vi "Append Strings to Log Control.vi"(8 "エラー入力 (エラーなし)":errorcluster, 10 "Appending Strings":string, 11 "Result Log Reference":refnum<vi>) -> (0 "エラー出力":errorcluster, 3 "Result Log Reference Out":refnum<vi>)   [LabVIEW 2020]
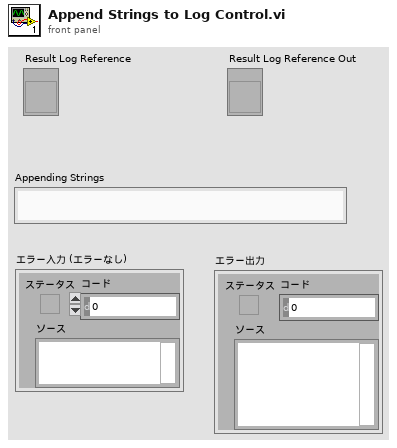
[diagram p1: front panel]
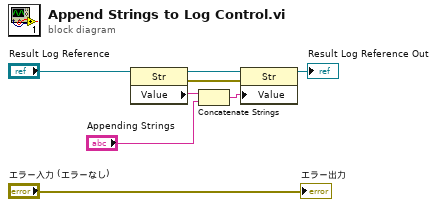
[diagram p0: block diagram]
diagram:
  n1 = property class="Str"(reference="Result Log Reference") -> (reference out=w3:refnum<vi>, error out=w2:errorcluster, "Value"=w5:string)  [unwired: 1 in]
  n2 = Concatenate Strings(w5, "Appending Strings") -> (w4:string)
  n3 = property class="Str"(reference=w3, error in=w2, "Value"=w4) -> (reference out=→"Result Log Reference Out":refnum<vi>)  [unwired: 1 out]
  "エラー出力" <- "エラー入力 (エラーなし)"
